vi "Day05-01_글로벌 변수(FGV).vi"() -> ()   [LabVIEW 2021]
panel:
  in  "불리언":bool
  out "결과값":dbl
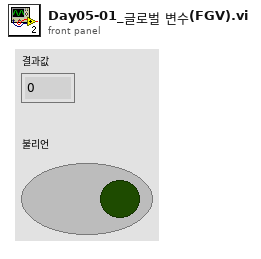
[diagram p1: front panel]
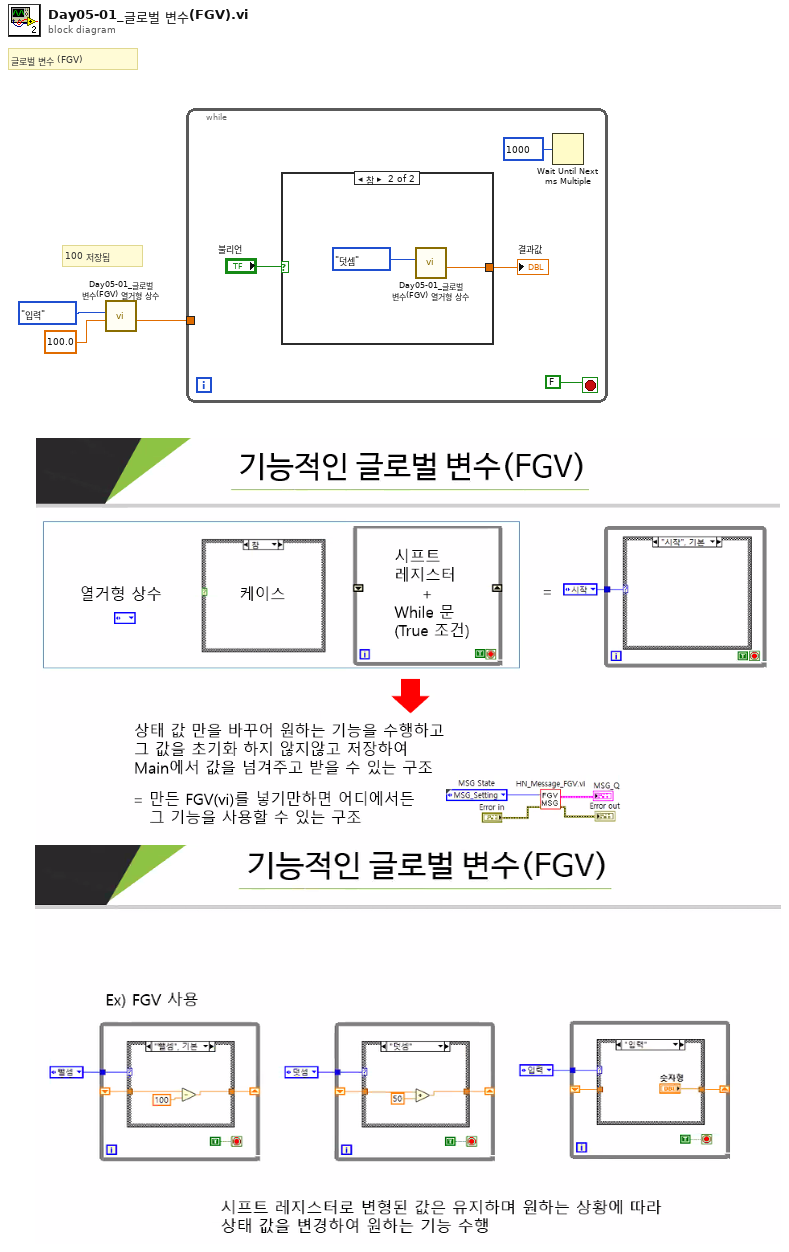
[diagram p0: block diagram]
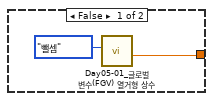
[diagram p2: hidden frame]
diagram:
  # "글로벌 변수 (FGV)"
  # "100 저장됨"
  n1 = call "Day05-01_글로벌 변수(FGV) 열거형 상수.vi"("숫자형"=100.0, "열거형"=enum16{"뺄셈", "덧셈", "입력"}."입력") -> ("결과값"=w2:dbl)  [unwired: 9 in]
  n2 = while {
    tunnel: w2 -> [_]
    stop <- FALSE stop-if-true
    n3 = case shown="참" "불리언" {
      tunnel: [w8 w10] -> w5
      frame False {
        n4 = call "Day05-01_글로벌 변수(FGV) 열거형 상수.vi"("열거형"=enum16{"뺄셈", "덧셈", "입력"}."뺄셈") -> ("결과값"=w8:dbl)  [unwired: 10 in]
      }
      frame True {
        n5 = call "Day05-01_글로벌 변수(FGV) 열거형 상수.vi"("열거형"=enum16{"뺄셈", "덧셈", "입력"}."덧셈") -> ("결과값"=w10:dbl)  [unwired: 10 in]
      }
    }
    "결과값" <- w5
    n6 = Wait Until Next ms Multiple(millisecond multiple=u32 1000 ("ms 배수")) -> ()  [unwired: 1 out]
  }
